vi "Set SR Cluster Item Visibility.vi"(8 "error in":errorcluster, 10 "Screen Width":i16, 11 "SR List ref in":refnum<vi>) -> (0 "error out":errorcluster)   [LabVIEW 2018]
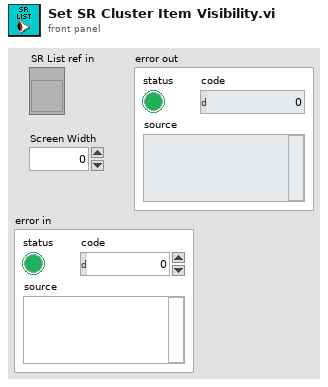
[diagram p1: front panel]
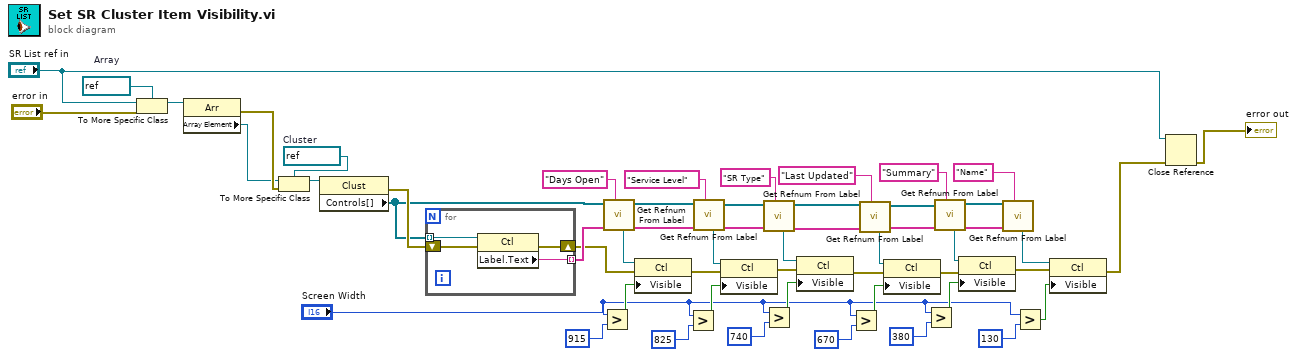
[diagram p0: block diagram]
diagram:
  w54 = refnum<vi> refnum  # Cluster
  w50 = refnum<vi> refnum  # Array
  n1 = To More Specific Class(target class=w50, reference="SR List ref in", error in="error in") -> (specific class reference=w51:refnum<vi>)  [unwired: 1 out]
  n2 = property class="Arr"(reference=w51) -> (error out=w53:errorcluster, "Array Element"=w52:refnum<vi>)  [unwired: 1 in, 1 out]
  n3 = To More Specific Class(target class=w54, reference=w52, error in=w53) -> (specific class reference=w9:refnum<vi>)  [unwired: 1 out]
  n4 = property class="Clust"(reference=w9) -> (error out=w10:errorcluster, "Controls[]"=w3:refnum<vi>[])  [unwired: 1 in, 1 out]
  n5 = for {
    tunnel: w3 -> [w56] mode=indexing
    shift-right: [w57] -> w1
    shift-left: w10 -> [w58]
    tunnel: [w55] -> w2 mode=indexing
    n6 = property class="Ctl"(reference=w56, error in=w58) -> (error out=w57:errorcluster, "Label.Text"=w55:string)  [unwired: 1 out]
  }
  n7 = Greater?(x="Screen Width", y=i16 915) -> (0:w39:bool)
  n8 = call "Get Refnum From Label.vi"("label"="Days Open", "label array in"=w2, "controls[] in"=w3) -> ("label array out"=w14:string[], "controls[] out"=w13:refnum<vi>[], "refnum out"=w44:refnum<vi>)  [unwired: 6 in]
  n9 = property class="Ctl"(reference=w44, error in=w1, "Visible"=w39) -> (error out=w41:errorcluster)  [unwired: 1 out]
  n10 = Greater?(x="Screen Width", y=i16 825) -> (0:w38:bool)
  n11 = call "Get Refnum From Label.vi"("label"="Service Level", "label array in"=w14, "controls[] in"=w13) -> ("label array out"=w15:string[], "controls[] out"=w16:refnum<vi>[], "refnum out"=w45:refnum<vi>)  [unwired: 6 in]
  n12 = property class="Ctl"(reference=w45, error in=w41, "Visible"=w38) -> (error out=w43:errorcluster)  [unwired: 1 out]
  n13 = call "Get Refnum From Label.vi"("label"="SR Type", "label array in"=w15, "controls[] in"=w16) -> ("label array out"=w19:string[], "controls[] out"=w18:refnum<vi>[], "refnum out"=w46:refnum<vi>)  [unwired: 6 in]
  n14 = Greater?(x="Screen Width", y=i16 740) -> (0:w35:bool)
  n15 = property class="Ctl"(reference=w46, error in=w43, "Visible"=w35) -> (error out=w42:errorcluster)  [unwired: 1 out]
  n16 = Greater?(x="Screen Width", y=i16 670) -> (0:w33:bool)
  n17 = call "Get Refnum From Label.vi"("label"="Last Updated", "label array in"=w19, "controls[] in"=w18) -> ("label array out"=w23:string[], "controls[] out"=w22:refnum<vi>[], "refnum out"=w47:refnum<vi>)  [unwired: 6 in]
  n18 = property class="Ctl"(reference=w47, error in=w42, "Visible"=w33) -> (error out=w34:errorcluster)  [unwired: 1 out]
  n19 = Greater?(x="Screen Width", y=i16 380) -> (0:w29:bool)
  n20 = call "Get Refnum From Label.vi"("label"="Summary", "label array in"=w23, "controls[] in"=w22) -> ("label array out"=w25:string[], "controls[] out"=w24:refnum<vi>[], "refnum out"=w31:refnum<vi>)  [unwired: 6 in]
  n21 = property class="Ctl"(reference=w31, error in=w34, "Visible"=w29) -> (error out=w48:errorcluster)  [unwired: 1 out]
  n22 = call "Get Refnum From Label.vi"("label"="Name", "label array in"=w25, "controls[] in"=w24) -> ("refnum out"=w49:refnum<vi>)  [unwired: 6 in, 2 out]
  n23 = Greater?(x="Screen Width", y=i16 130) -> (0:w28:bool)
  n24 = property class="Ctl"(reference=w49, error in=w48, "Visible"=w28) -> (error out=w7:errorcluster)  [unwired: 1 out]
  n25 = Close Reference(reference="SR List ref in", error in (no error)=w7) -> (error out=→"error out":errorcluster)
